vi "mod_control changed(single).vi"(2 "Ctl Refnum":refnum<vi>, 4 "initialize?":bool) -> (7 "changed?":bool)   [LabVIEW 2020, in "niAMT.lvlib"]
uses:
  <vilib>/addons/Modulation/niAMT.lvlib
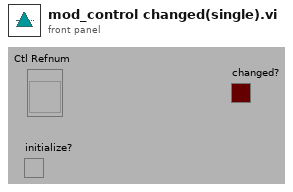
[diagram p1: front panel]
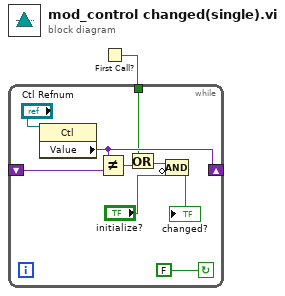
[diagram p0: block diagram]
diagram:
  n1 = First Call?() -> (First Call?: T/F=w1:bool)
  n2 = while {
    tunnel: w1 -> [w2]
    shift-left: _ -> [w4]
    shift-right: [w5] -> _
    stop <- FALSE continue-if-true
    n3 = property class="Ctl"(reference="Ctl Refnum") -> ("Value"=w5:variant)  [unwired: 1 in, 2 out]
    n4 = Not Equal?(x=w5, y=w4) -> (x != y?=w10:bool)
    n5 = Or(x=w2, y=w10) -> (x .or. y?=w3:bool)
    n6 = Compound Arithmetic op=AND(w3, invert "initialize?") -> (→"changed?":bool)
  }
